vi "PZC_MoveAbs.vi"(3 "error in":errorcluster, 4 "Target":dbl, 5 "Instrument":string) -> (0 "error out":errorcluster, 1 "Final Position":i32, 2 "Instrument out":string)   [LabVIEW 2019]
panel:
  out "Current Position":i32
  out "Command":string
  out "Move relative":dbl
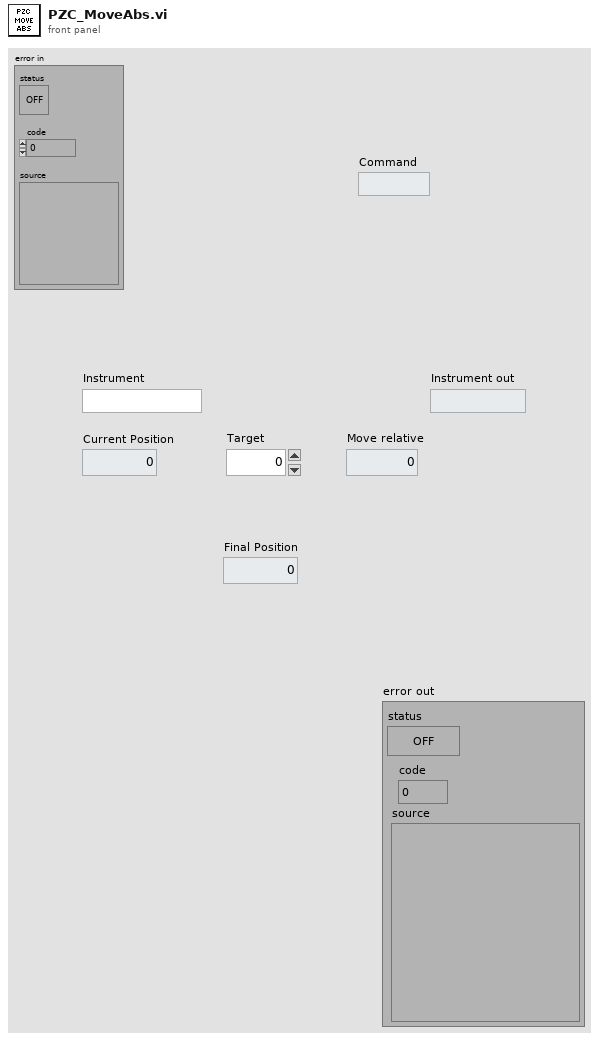
[diagram p1: front panel]
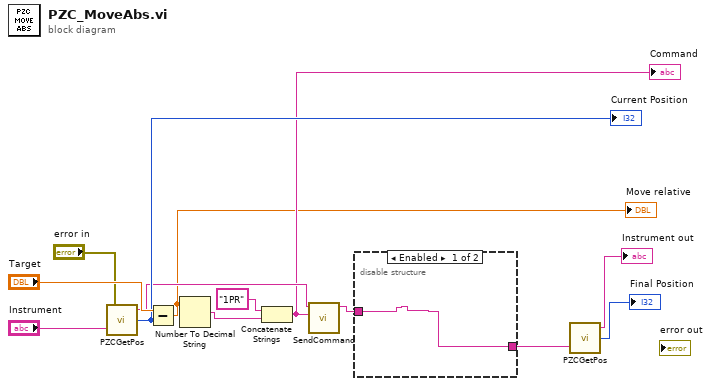
[diagram p0: block diagram]
diagram:
  n1 = call "PZCGetPos.vi"("error in"="error in", "Instrument Channel"="Instrument") -> ("Instrument Channel Out"=w10:string, "Position"=w11:i32)  [unwired: 1 out]
  "Current Position" <- w11
  n2 = Subtract(x="Target", y=w11) -> (x-y=w5:dbl)
  "Move relative" <- w5
  n3 = Number To Decimal String(number=w5) -> (decimal integer string=w8:string)  [unwired: 1 in]
  n4 = Concatenate Strings("1PR", w8) -> (w7:string)
  "Command" <- w7
  n5 = call "SendCommand.vi"("Command"=w7, "Instrument Channel"=w10) -> ("Instrument Channel out"=w3:string)  [unwired: 8 in, 1 out]
  n6 = disable-structure shown="Enabled" {
    disable-tunnel: w3 -> [w14 w15]
    disable-tunnel: [w14 w15] -> w2
    frame Enabled {
    }
    frame Disabled {
    }
  }
  n7 = call "PZCGetPos.vi"("Instrument Channel"=w2) -> ("Instrument Channel Out"=→"Instrument out":string, "Position"=→"Final Position":i32)  [unwired: 1 in, 1 out]
